vi "Async Methods Actor.vi"() -> ()   [LabVIEW 2021, in "Async Methods Actor.lvlib"]
uses:
  Async Methods Actor.lvlib
  Async Methods Actor/Async Methods Actor.lvclass
panel:
  in  "Async Methods Actor":refnum<class "Async Methods Actor.lvclass">
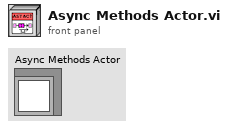
[diagram p1: front panel]
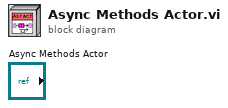
[diagram p0: block diagram]
diagram:
